vi "CalcParams.vi"(0 "ClkRate":dbl[unit] format="%#_6p", 5 "fc":dbl[unit] format="%#_6p", 7 "Deadtime":dbl[unit] format="%#_6p") -> (4 "Parameters":T1={"FreqCarrier"=0, "DeadtimeTicks"=1, "TriangleInc"=0.0})   [LabVIEW 2015, in "SPWMInterface.lvlib"]
doc: "Calculates parameters nescessary to configure the SPWM Core.\n\nClkRate - The clock rate in Hz that the core will execute at, typically determined by the clock rate of a single cycle timed loop. Typical values would be 40 MHz or 80 MHz. Recommended values would be 10 to 20 kHz.\n\nfc - Carrier frequency in Hz of the PWM. Recommended values would be 10 kHz to 20 kHz.\n\nDeadtime - Deadtime between switching between the Top and Bottom switch pairs in seconds."
uses:
  SPWMInterface.lvlib
  SPWM/SwitchConfig.ctl
  SPWM/SPWM.lvlib
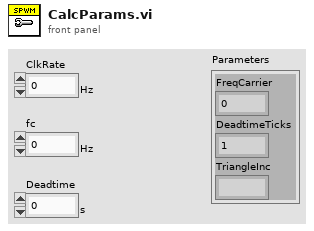
[diagram p1: front panel]
types:
  T1 = typedef "SPWM.lvlib/SwitchConfig.ctl" = cluster{"FreqCarrier":u32, "DeadtimeTicks":u8, "TriangleInc":fxp<+/-,32,4>}
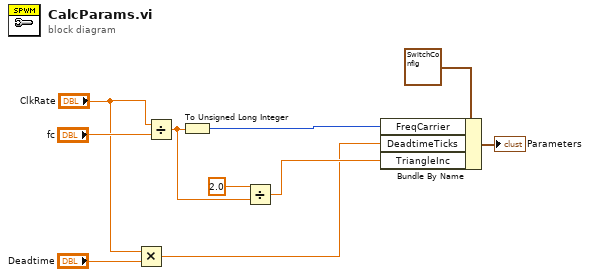
[diagram p0: block diagram]
diagram:
  n1 = Multiply(x="ClkRate", y="Deadtime") -> (x*y=w2:dbl)
  n2 = Divide(x="ClkRate", y="fc") -> (x/y=w6:dbl)
  n3 = To Unsigned Long Integer(number=w6) -> (unsigned 32bit integer=w8:u32)
  n4 = Divide(x=2.0, y=w6) -> (x/y=w5:dbl)
  n5 = Bundle By Name(cluster=T1 {"FreqCarrier"=0, "DeadtimeTicks"=1, "TriangleInc"=0.0} ("SwitchConfig"), "FreqCarrier"=w8, "DeadtimeTicks"=w2, "TriangleInc"=w5) -> (→"Parameters":T1)
